vi "test Set ObjectType_2.vi"(11 "Test Case In":refnum<class "test EDS.lvclass">) -> (0 "error out":errorcluster, 3 "Test Case Out":refnum<class "test EDS.lvclass">)   [LabVIEW 2024, in "test EDS.lvclass"]
uses:
  test EDS.lvclass
  C:/Program Files/National Instruments/LabVIEW 2024/vi.lib/Astemes/LUnit/Test Case.lvclass
  <vilib>/PNR/JSONtext Object Serialization/Generic Object Serializer/Generic Object Serializer.lvclass
  C:/Program Files/National Instruments/LabVIEW 2024/vi.lib/JDP Science/JSONtext/LVClass Serializer/JSONtext LVClass Serializer.lvclass
  <vilib>/PNR/JSONtext Object Serialization/Generic Object Serializer/Type Name Handling.ctl
  Core/Object Type/Object Type Base.lvclass
  <vilib>/PNR/JSONtext Object Serialization/Generic Object Serializer/Generic Object Serializer.lvclass/Generic Object Serializer.ctl
  <vilib>/Astemes/LUnit/Test Case.lvclass/Test Case.ctl
  bdd25f00-0f07-479c-b713-0b173a884aa2.vi
  9c146d8d-ecb2-4a43-97e4-092ef5af0c10.vi
  <vilib>/PNR/JSONtext Object Serialization/Generic Object Serializer/Write Type Name Handling.vi
  <vilib>/Astemes/LUnit/Append Fail Result.vi
  <vilib>/Astemes/LUnit/Append Pass Result.vi
  <vilib>/Astemes/LUnit/Describe Comparison.vi
  9c146d8d-ecb2-4a43-97e4-092ef5af0c10.vi/4479f1b4-f4e5-41cd-8a07-3589632eefcf.vi
  <vilib>/Astemes/LUnit/Run In UI.vi
  <vilib>/Utility/error.llb/Clear Errors.vi
  <vilib>/JDP Science/JSONtext/Variant to JSON Text.vi
  <vilib>/Astemes/LUnit/Describe Variant.vi
  test EDS.lvclass/test EDS.ctl
  Core/Value/Value.lvclass
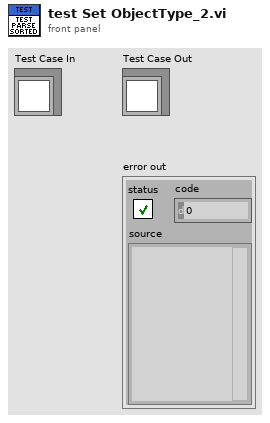
[diagram p1: front panel]
types:
  T1 = typedef "Generic Object Serializer.lvclass/Type Name Handling.ctl" = enum16{"None", "Inline"}
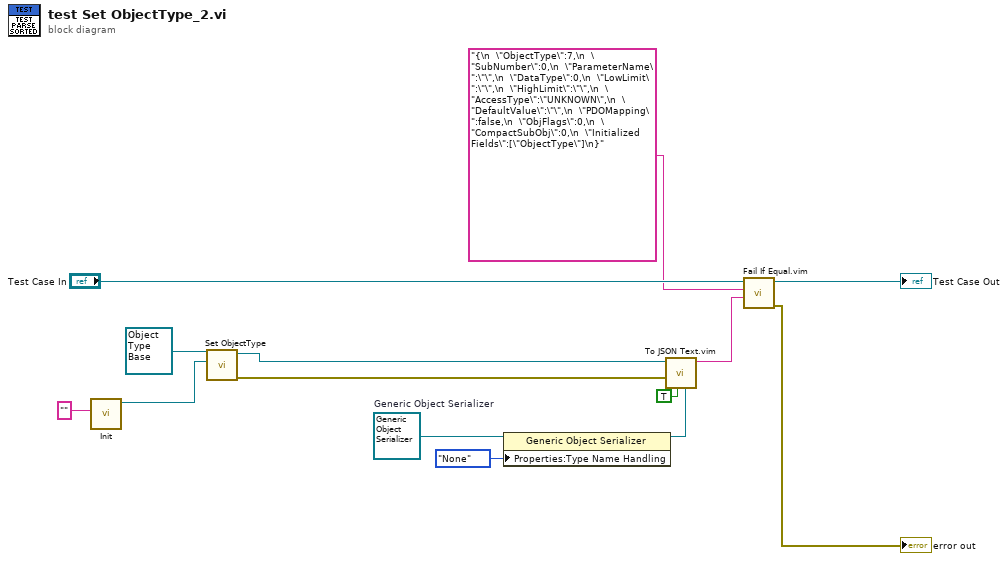
[diagram p0: block diagram]
diagram:
  w11 = refnum<class "Generic Object Serializer.lvclass"> refnum  # Generic Object Serializer
  n1 = call "Init.vi"("Value"="") -> ("Value out"=w5:refnum<class "Value.lvclass">)  [unwired: 9 in, 1 out]
  n2 = call-dynamic "Set ObjectType.vi"("ObjectType"=w5, "Object Type in"=refnum<class "Object Type Base.lvclass"> refnum ("EDS.lvlib:Object Type.lvclass")) -> ("error out"=w2:errorcluster, "Object Type out"=w3:refnum<class "Object Type Base.lvclass">)  [unwired: 8 in]
  n3 = property class="Generic Object Serializer"(reference=w11, "Properties:Type Name Handling"=Type_Name_Handling."None" ("Type Name Handling")) -> (reference out=w10:refnum<class "Generic Object Serializer.lvclass">)  [unwired: 1 in, 1 out]
  n4 = call "To JSON Text.vim"("LVClass Serializer"=w10, "Pretty Print?"=TRUE, "error in (no error)"=w2, "Anything"=w3) -> ("<JSON>"=w7:string)  [unwired: 6 in, 1 out]
  n5 = call "Fail If Equal.vim"("Actual"=w7, "Unexpected"="{\n  \"ObjectType\":7,\n  \"SubNumber\":0,\n  \"ParameterName\":\"\",\n  \"DataType\":0,\n  \"LowLimit\":\"\",\n  \"HighLimit\":\"\",\n  \"AccessType\":\"UNKNOWN\",\n  \"DefaultValue\":\"\",\n  \"PDOMapping\":false,\n  \"ObjFlags\":0,\n  \"CompactSubObj\":0,\n  \"Initialized Fields\":[\"ObjectType\"]\n}" ("<JSON> 2"), "LUnit Test Case In"="Test Case In") -> ("error out"=→"error out":errorcluster, "LUnit Test Case Out"=→"Test Case Out":refnum<class "test EDS.lvclass">)  [unwired: 7 in]
